vi "GetPercentage.vi"(8 "total number":i32, 11 "current number":i32) -> (1 "percentage":dbl)   [LabVIEW 2022 SP3]
doc: "This VI derives a percentage.\n\nInputs :\n- The current number (I32)\n- The total number (I32)\n\nOutput :\n- The percentage (DBL)"
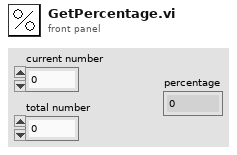
[diagram p1: front panel]
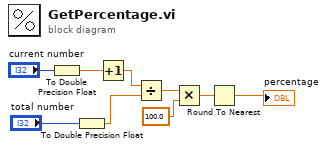
[diagram p0: block diagram]
diagram:
  n1 = To Double Precision Float(number="current number") -> (double precision float=w9:dbl)
  n2 = To Double Precision Float(number="total number") -> (double precision float=w1:dbl)
  n3 = Increment(x=w9) -> (x+1=w2:dbl)
  n4 = Divide(x=w2, y=w1) -> (x/y=w6:dbl)
  n5 = Multiply(x=w6, y=100.0) -> (x*y=w8:dbl)
  n6 = Round To Nearest(number=w8) -> (nearest integer value=→"percentage":dbl)
